vi "Interface_Asset_Map Status.vi"(8 "error in (no error)":errorcluster, 11 "Grid_Virtual in":refnum<class "Grid_Virtual.lvclass">) -> (0 "error out":errorcluster, 3 "Grid_Virtual out":refnum<class "Grid_Virtual.lvclass">)   [LabVIEW 2015, in "Grid_Virtual.lvclass"]
uses:
  Grid_Virtual.lvclass
  Grid_Status.ctl
  Grid.lvclass
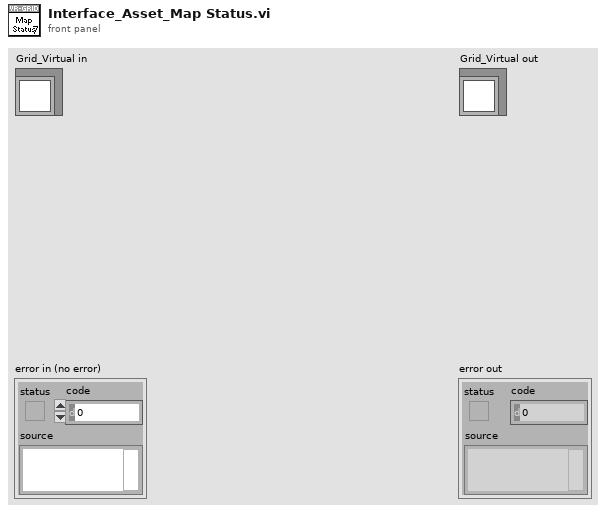
[diagram p1: front panel]
types:
  T1 = typedef "Grid.lvclass/Grid_Status.ctl" = cluster{"kW":dbl}
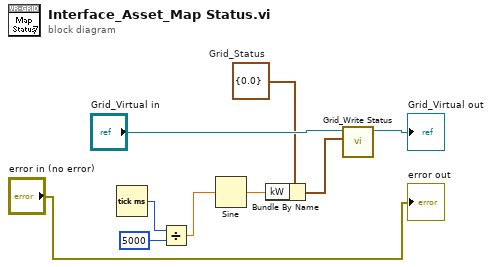
[diagram p0: block diagram]
diagram:
  w6 = T1 {"kW"=0.0}  # Grid_Status
  n1 = Tick Count (ms)() -> (millisecond timer value=w5:u32)
  n2 = Divide(x=w5, y=u32 5000) -> (x/y=w3:dbl)
  n3 = Sine(x=w3) -> (sin(x)=w2:dbl)
  n4 = Bundle By Name(cluster=w6, "kW"=w2) -> (w7:T1)
  n5 = call-dynamic "Grid_Write Status.vi"("Grid_Status"=w7, "Grid in"="Grid_Virtual in") -> ("Grid out"=→"Grid_Virtual out":refnum<class "Grid_Virtual.lvclass">)  [unwired: 9 in]
  "error out" <- "error in (no error)"
